vi "_Check ADCs.vi"(4 "ADC Table":T1[](array[typedef]), 5 "ADC Values":i32[](array[numeric]), 7 "ADC List Ref":refnum<vi>) -> (3 "Interlocks":bool[](array[boolean]))   [LabVIEW 2015]
uses:
  Type/_RT Configuration 2.ctl
  Configuration/_Global Configuration.vi
panel:
  out "DoorOK":bool
  out "VacRdy":bool
  out "HG1OK":bool
  out "HG2OK":bool
  out "DryingGasOK":bool
  out "ExhaustOK":bool
  out "SourceOK":bool
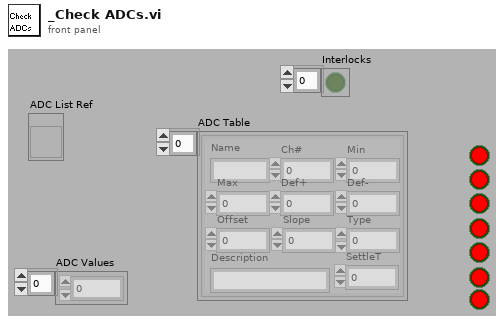
[diagram p1: front panel]
types:
  T1 = typedef "_RT Configuration 2.ctl" = cluster{"Name":string, "Ch#":u8, "Min":dbl, "Max":dbl, "Def+":dbl, "Def-":dbl, "Offset":dbl, "Slope":dbl, "Type":u8, "Description":string, "SettleT":dbl}
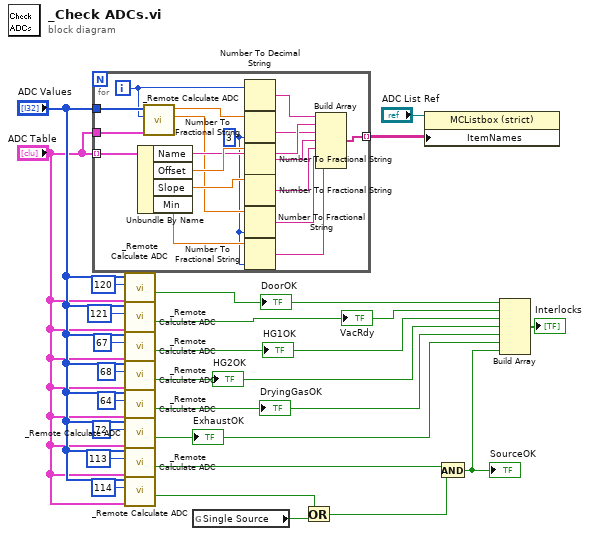
[diagram p0: block diagram]
diagram:
  n1 = for {
    tunnel: "ADC Values" -> [w42]
    tunnel: "ADC Table" -> [w40] mode=indexing
    tunnel: "ADC Table" -> [w41]
    tunnel: [w32] -> w23 mode=indexing
    i -> [w31]
    w25 = i16 3 ("precision (6)")
    n2 = Unbundle By Name(w40) -> ("Name"=w36:string, "Offset"=w39:dbl, "Slope"=w38:dbl, "Min"=w26:dbl)
    n3 = call "_Remote Calculate ADC.vi"("ADC Table"=w41, "ADC Channel (64)"=w31, "ADC Values"=w42) -> ("User Value"=w29:dbl, "Raw Reading"=w30:dbl)  [unwired: 1 in, 2 out]
    n4 = Number To Decimal String(number=w31) -> (decimal integer string=w37:string)  [unwired: 1 out]
    n5 = Number To Fractional String(number=w30, precision (6)=w25) -> (F-format string=w35:string)  [unwired: 2 out]
    n6 = Number To Fractional String(number=w39) -> (F-format string=w34:string)  [unwired: 3 out]
    n7 = Number To Fractional String(number=w38) -> (F-format string=w33:string)  [unwired: 3 out]
    n8 = Number To Fractional String(number=w29, precision (6)=w25) -> (F-format string=w28:string)  [unwired: 2 out]
    n9 = Number To Fractional String(number=w26, precision (6)=w25) -> (F-format string=w27:string)  [unwired: 2 out]
    n10 = Build Array(w37, w36, w35, w34, w33, w28, w27) -> (w32:string[])
  }
  n11 = call "_Remote Calculate ADC.vi"("ADC Table"="ADC Table", "ADC Channel (64)"=u8 120, "ADC Values"="ADC Values") -> ("In Range?"=w5:bool)  [unwired: 1 in, 3 out]
  "DoorOK" <- w5
  n12 = call "_Remote Calculate ADC.vi"("ADC Table"="ADC Table", "ADC Channel (64)"=u8 121, "ADC Values"="ADC Values") -> ("In Range?"=w6:bool)  [unwired: 1 in, 3 out]
  "VacRdy" <- w6
  n13 = call "_Remote Calculate ADC.vi"("ADC Table"="ADC Table", "ADC Channel (64)"=u8 67, "ADC Values"="ADC Values") -> ("In Range?"=w12:bool)  [unwired: 1 in, 3 out]
  "HG1OK" <- w12
  n14 = call "_Remote Calculate ADC.vi"("ADC Table"="ADC Table", "ADC Channel (64)"=u8 68, "ADC Values"="ADC Values") -> ("In Range?"=w11:bool)  [unwired: 1 in, 3 out]
  "HG2OK" <- w11
  n15 = call "_Remote Calculate ADC.vi"("ADC Table"="ADC Table", "ADC Channel (64)"=u8 64, "ADC Values"="ADC Values") -> ("In Range?"=w10:bool)  [unwired: 1 in, 3 out]
  "DryingGasOK" <- w10
  n16 = call "_Remote Calculate ADC.vi"("ADC Table"="ADC Table", "ADC Channel (64)"=u8 72, "ADC Values"="ADC Values") -> ("In Range?"=w9:bool)  [unwired: 1 in, 3 out]
  "ExhaustOK" <- w9
  n17 = call "_Remote Calculate ADC.vi"("ADC Table"="ADC Table", "ADC Channel (64)"=u8 113, "ADC Values"="ADC Values") -> ("In Range?"=w4:bool)  [unwired: 1 in, 3 out]
  n18 = call "_Remote Calculate ADC.vi"("ADC Table"="ADC Table", "ADC Channel (64)"=u8 114, "ADC Values"="ADC Values") -> ("In Range?"=w2:bool)  [unwired: 1 in, 3 out]
  n19 = global read "_Global Configuration.vi" "Single Source"() -> (w3:bool)
  n20 = Or(x=w2, y=w3) -> (x .or. y?=w1:bool)
  n21 = property class="MCListbox (strict)"(reference="ADC List Ref", "ItemNames"=w23) -> ()  [unwired: 1 in, 2 out]
  n22 = And(x=w4, y=w1) -> (x .and. y?=w8:bool)
  "SourceOK" <- w8
  n23 = Build Array(w5, w6, w12, w11, w10, w9, w8) -> (→"Interlocks":bool[])
